vi "Export.vi"(8 "error in (no error)":errorcluster, 9 "Items":refnum<class "ILabVIEWItem.lvclass">[](array[class]), 11 "CGrapherDGML in":refnum<class "CGrapherDGML.lvclass">) -> (0 "error out":errorcluster, 3 "CGrapherDGML out":refnum<class "CGrapherDGML.lvclass">)   [LabVIEW 2020, in "DefaultExtensions.lvlib" / "CGrapherDGML.lvclass"]
uses:
  CGrapherDGML.lvclass
  obj/Addons/LabVIEWObjectInterfaces.lvlibp/LabVIEWObjectInterfaces/ILabVIEWItem/ILabVIEWItem.lvclass
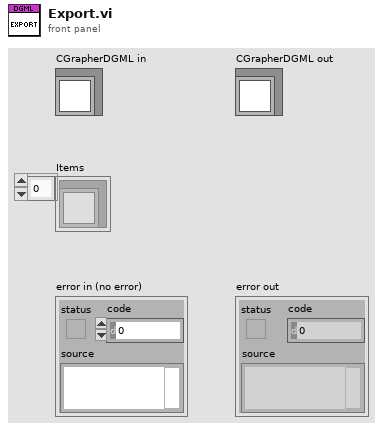
[diagram p1: front panel]
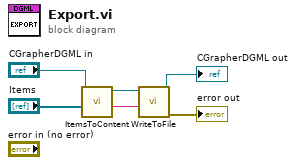
[diagram p0: block diagram]
diagram:
  n1 = call-dynamic "ItemsToContent.vi"("Items"="Items", "CGrapherDGML in"="CGrapherDGML in") -> ("Export string"=w2:string, "CGrapherDGML out"=w3:refnum<class "CGrapherDGML.lvclass">)  [unwired: 7 in, 1 out]
  n2 = call-dynamic "WriteToFile.vi"("Export string"=w2, "CGrapherDGML in"=w3) -> ("error out"=→"error out":errorcluster, "CGrapherDGML out"=→"CGrapherDGML out":refnum<class "CGrapherDGML.lvclass">)  [unwired: 8 in]
